vi "myRIO_BRig_RT_comm_webdav_uploadReceived_read.vi"(9 "input_dataSize":i32, 11 "input_filePath":path) -> (1 "output_Ivalid":bool, 3 "output_data":i64[](array[numeric]))   [LabVIEW 2014]
uses:
  <vilib>/Utility/file.llb/Read From Spreadsheet File (I64).vi
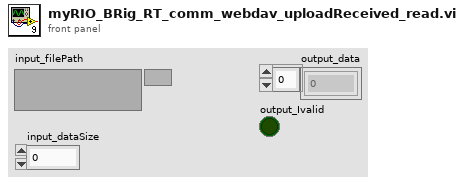
[diagram p1: front panel]
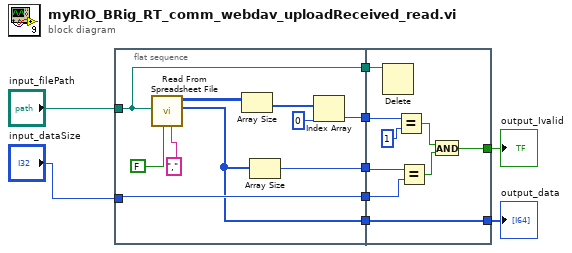
[diagram p0: block diagram]
diagram:
  n1 = flat-sequence {
    tunnel: "input_filePath" -> [w14]
    tunnel: [w14] -> w8
    tunnel: [w13] -> w7
    tunnel: [w12] -> w6
    tunnel: "input_dataSize" -> [w11]
    tunnel: [w11] -> w5
    tunnel: [w10] -> w3
    tunnel: w8 -> [w28]
    tunnel: w7 -> [w26]
    tunnel: w6 -> [w25]
    tunnel: w5 -> [w24]
    tunnel: [w21] -> w1
    tunnel: w3 -> [w20]
    tunnel: [w20] -> w2
    frame #0 {
      n2 = call-poly <vilib>:"Read From Spreadsheet File.vi"("delimiter (\\t)"="," ("delimiter (\\t)"), "transpose (no:F)"=FALSE, "file path (dialog if empty)"=w14) -> ("first row"=w10:i64[], "all rows"=w17:i64[][])  [unwired: 4 in, 3 out]
      n3 = Array Size(array=w17) -> (size(s)=w16:i32[])
      n4 = Array Size(array=w10) -> (size(s)=w12:i32)
      n5 = Index Array(array=w16, index=0) -> (element=w13:i32)
    }
    frame #1 {
      n6 = Delete(path (use dialog)=w28) -> ()  [unwired: 4 in, 3 out]
      n7 = Equal?(x=w26, y=1) -> (x = y?=w22:bool)
      n8 = Equal?(x=w25, y=w24) -> (x = y?=w23:bool)
      n9 = And(x=w22, y=w23) -> (x .and. y?=w21:bool)
    }
  }
  "output_data" <- w2
  "output_Ivalid" <- w1
